vi "Write Cycle Time (ms).vi"(8 "error in (no error)":errorcluster, 10 "Cycle Time (ms)":u32, 11 "Query in":refnum<class "Query.lvclass">) -> (0 "error out":errorcluster, 3 "Query out":refnum<class "Query.lvclass">)   [LabVIEW 2018, in "Query.lvclass"]
doc: "Query.lvclass:Write Cycle Time.vi\n\nThis VI is the accessor for writing the Cycle Time parameter for the Query class.\n\nInstrument Communication Module Version 1.0\nDecember, 2017 Original Code Consulting David Thomson\n www.originalcode.com"
uses:
  Query.lvclass
  Query.lvclass/Query.ctl
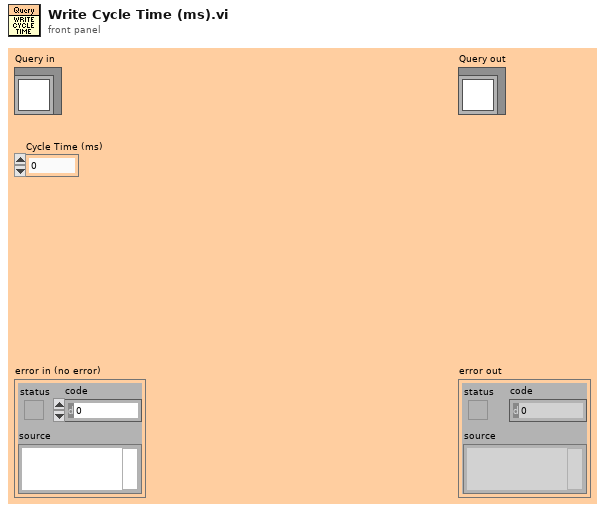
[diagram p1: front panel]
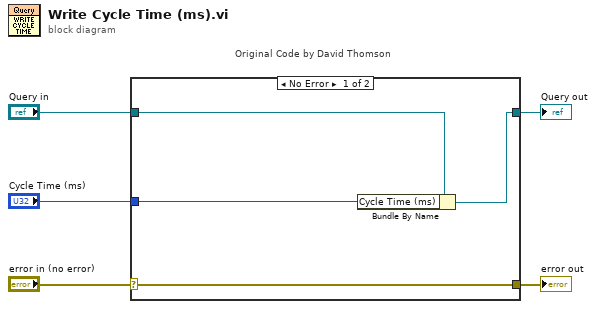
[diagram p0: block diagram]
diagram:
  n1 = case "Original Code by David Thomson" shown="No Error" "error in (no error)" {
    selector: "error in (no error)" -> [w9 w10]
    tunnel: [w9 w10] -> w4
    tunnel: [w7 w11] -> w2
    tunnel: "Query in" -> [w8 w11]
    tunnel: "Cycle Time (ms)" -> [w6 _]
    frame No Error {
      n2 = Bundle By Name(cluster=w8, "Cycle Time (ms)"=w6) -> (w7:refnum<class "Query.lvclass">)
    }
    frame Error {
    }
  }
  "error out" <- w4
  "Query out" <- w2
